vi "NicmosController.vi"() -> ()   [LabVIEW 2009]
uses:
  Controls/NICMOS.MASKBANKS.ctl
  Controls/NICMOS.COMMANDBASIC.ctl
  Controls/NICMOS.STATE.ctl
  Controls/NICMOS.FILTERLIST.ctl
  Controls/NICMOS.FILTER.ctl
  Controls/NICMOS.COMMAND.ctl
  Controls/NICMOS.READOUT.ctl
  Controls/NICMOS.FILTERCOMMAND.ctl
  Controls/NICMOS.TEMPERATURE.ctl
  NicmosGlobal.vi
panel:
  out "ACQ":i32
  in  "FilterList":T1=["DARK1", "J", "DARK3", "H", "DARK5", "K'", "BrG", "K203", "K215", "K222", "K239", "DARK12"]
  out "error out":errorcluster
  out "Index":i32
  out "STATE":T3
  out "COMMANDBASIC":T4=enum."QUIT"
  in  "VISA":string="COM31"
  in  "PROCESS":string="NICMOS"
  in  "MaskBanks":T5=[{"MaskList"=[{"X"=6, "Y"=6, "NX"=1, "NY"=1}], "Reform X"=1, "Reform Y"=1}, {"MaskList"=[{"X"=2, "Y"=2, "NX"=9, "NY"=9}], "Reform X"=9, "Reform Y"=9}, {"MaskList"=[{"X"=48, "Y"=38, "NX"=1, "NY"=8}], "Reform X"=1, "Reform Y"=8}, {"MaskList"=[{"X"=44, "Y"=38, "NX"=8, "NY"=8}], "Reform X"=8, "Reform Y"=8}, {"MaskList"=[{"X"=14, "Y"=7, "NX"=35, "NY"=8}], "Reform X"=35, "Reform Y"=8}, {"MaskList"=[{"X"=2, "Y"=2, "NX"=100, "NY"=100}], "Reform X"=100, "Reform Y"=100}]
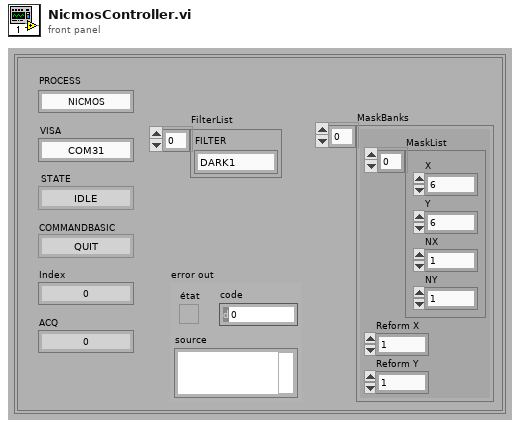
[diagram p1: front panel]
types:
  T1 = typedef "NICMOS.FILTERLIST.ctl" = T2[]
  T2 = typedef "NICMOS.FILTER.ctl" = string
  T3 = typedef "NICMOS.STATE.ctl" = enum16{"IDLE", "WRITING BANKS", "SETTING FILTER", "HOMING FILTER", "QUERYING TEMP", "CONFIGURING", "STARTING", "RUNNING", "HALTING", "STOPPED"}
  T4 = typedef "NICMOS.COMMANDBASIC.ctl" = enum16{"WRITE BANKS", "SET FILTER", "HOME FILTER", "QUERY TEMP", "CONFIGURE", "START", "ACQUISITION", "STOP", "QUIT"}
  T5 = typedef "NICMOS.MASKBANKS.ctl" = cluster{"MaskList":cluster{"X":i32, "Y":i32, "NX":i32, "NY":i32}[], "Reform X":i32, "Reform Y":i32}[]
  T6 = typedef "NicmosSynchronization.ctl" = cluster{"COMMAND":T7, "STATE":T8, "DATA":T9, "ACQUISITION":T10, "RAW":T11, "TEMPERATURE":T12, "READOUT":T13, "FILTER":T14, "MASKBANKS":T15}
  T7 = typedef "NICMOS.COMMAND.QUEUE.ctl" = refnum<queue>
  T8 = typedef "NICMOS.STATE.NOTIFIER.ctl" = refnum<notifier>
  T9 = typedef "NICMOS.DATA.NOTIFIER.ctl" = refnum<notifier>
  T10 = typedef "NICMOS.DATA.QUEUE.ctl" = refnum<queue>
  T11 = typedef "NICMOS.RAW.NOTIFIER.ctl" = refnum<notifier>
  T12 = typedef "NICMOS.TEMPERATURE.NOTIFIER.ctl" = refnum<notifier>
  T13 = typedef "NICMOS.READOUT.NOTIFIER.ctl" = refnum<notifier>
  T14 = typedef "NICMOS.FILTER.NOTIFIER.ctl" = refnum<notifier>
  T15 = typedef "NICMOS.MASKBANKS.NOTIFIER.ctl" = refnum<notifier>
  T16 = typedef "NICMOS.COMMAND.ctl" = cluster{"Command":T4, "READOUT":T17, "FILTERCOMMAND":T18, "ACQUISITION":i32, "Done":refnum<k4>}
  T17 = typedef "NICMOS.READOUT.ctl" = cluster{"Readout":i32, "Deglitch":i32, "Framerate":dbl[unit], "Bank":i32}
  T18 = typedef "NICMOS.FILTERCOMMAND.ctl" = cluster{"FILTER":T2, "INIT":bool}
  T19 = typedef "NICMOS.TEMPERATURE.ctl" = cluster{"T1":dbl, "T2":dbl}
  T20 = typedef "NICMOS.RAW.ctl" = u16[][][]
  T21 = typedef "NICMOS.DATA.ctl" = cluster{"DATA":i32[][][], "INDEX":i32}
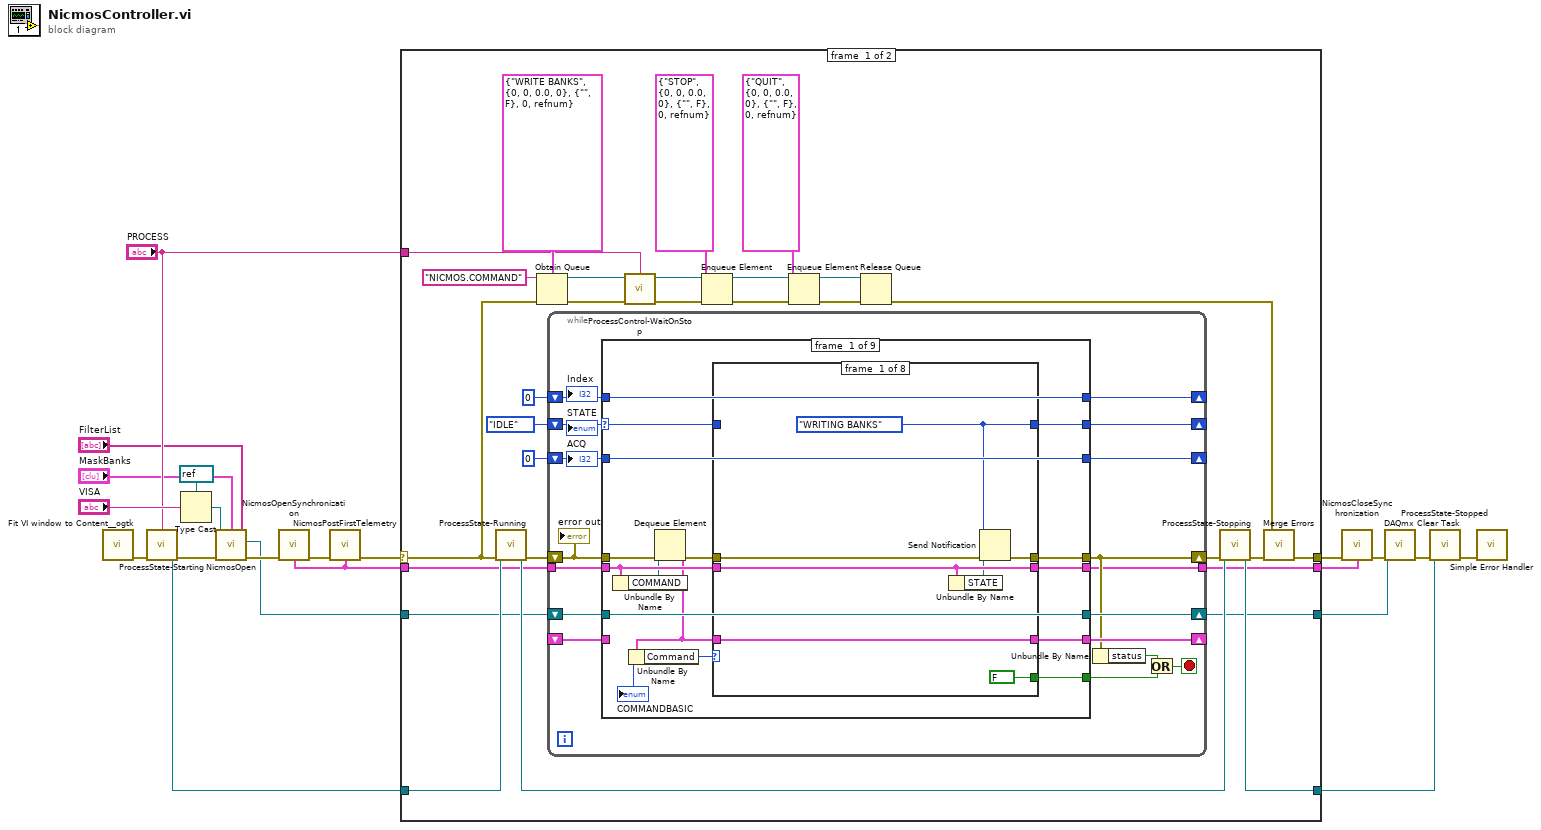
[diagram p0: block diagram]
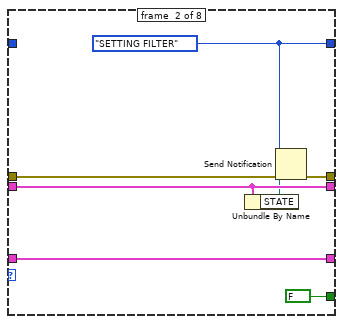
[diagram p2: hidden frame]
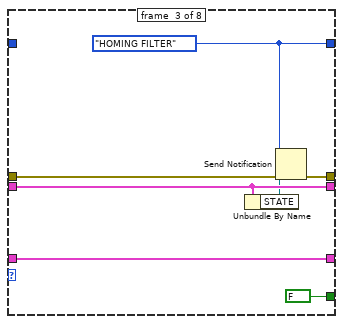
[diagram p3: hidden frame]
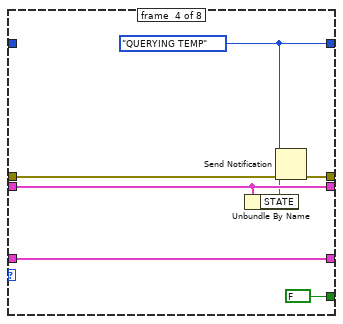
[diagram p4: hidden frame]
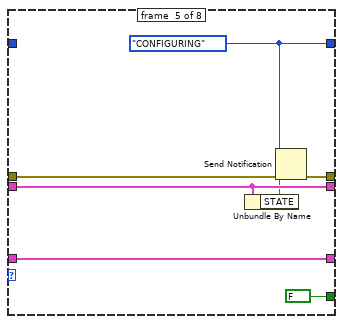
[diagram p5: hidden frame]
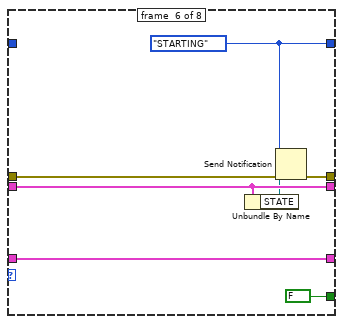
[diagram p6: hidden frame]
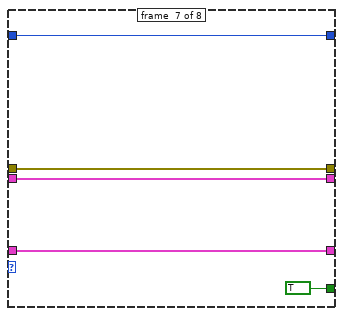
[diagram p7: hidden frame]
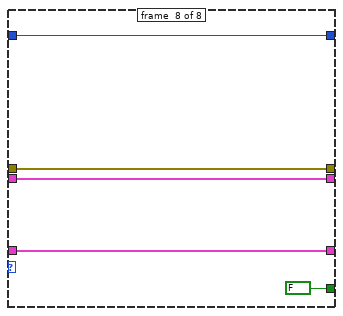
[diagram p8: hidden frame]
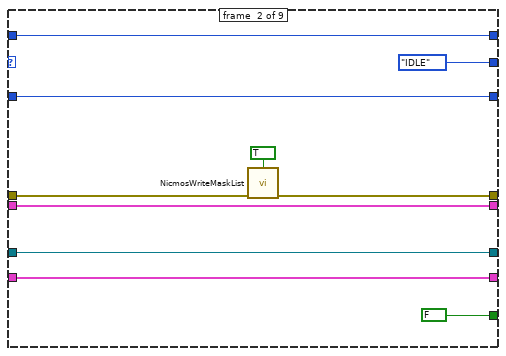
[diagram p9: hidden frame]
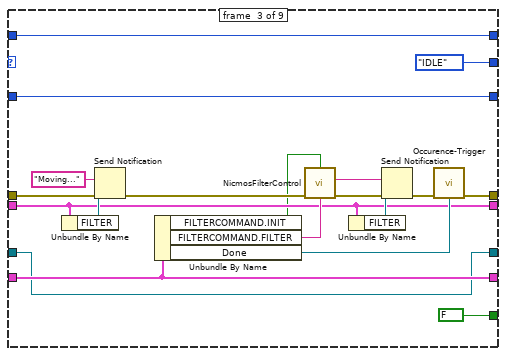
[diagram p10: hidden frame]
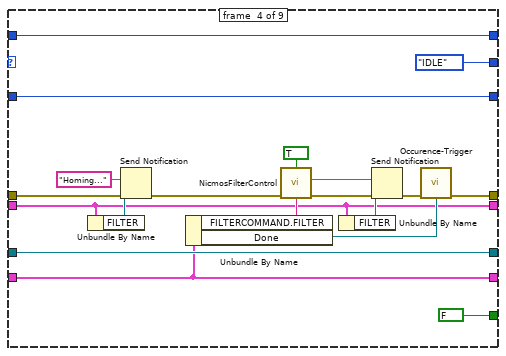
[diagram p11: hidden frame]
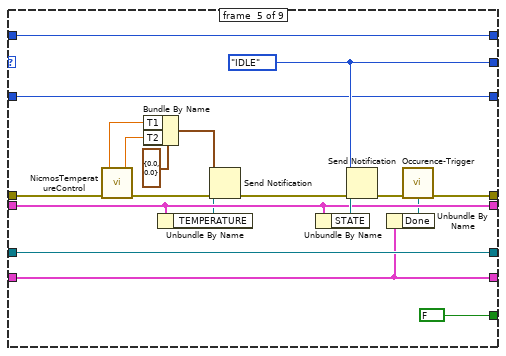
[diagram p12: hidden frame]
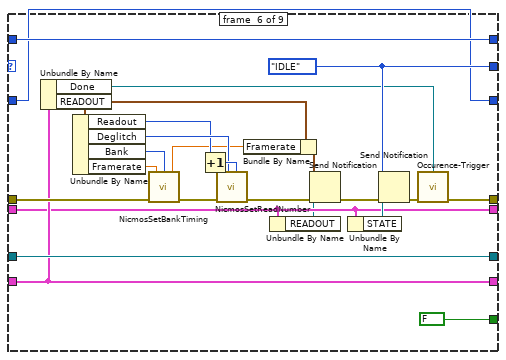
[diagram p13: hidden frame]
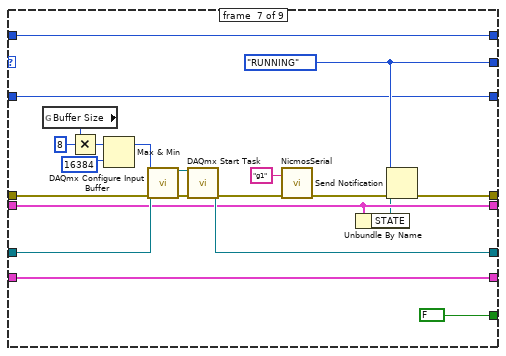
[diagram p14: hidden frame]
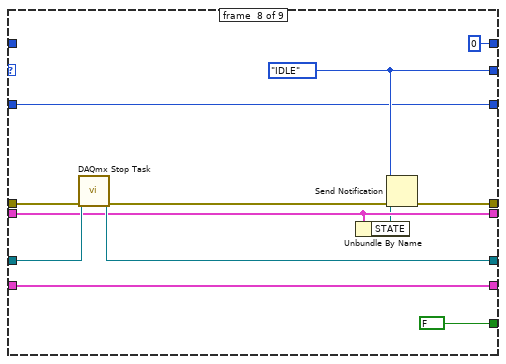
[diagram p15: hidden frame]
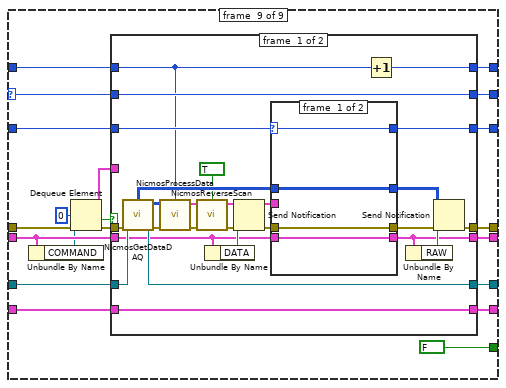
[diagram p16: hidden frame]
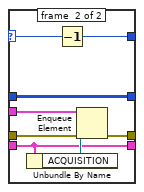
[diagram p17: hidden frame]
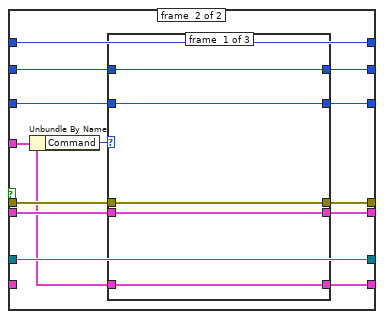
[diagram p18: hidden frame]
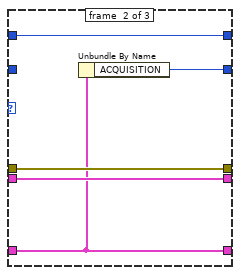
[diagram p19: hidden frame]
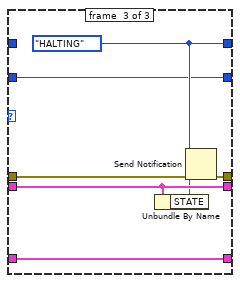
[diagram p20: hidden frame]
diagram:
  n1 = call <userlib>:"Fit VI window to Content__ogtk.vi"() -> ("error out"=w21:errorcluster)  [unwired: 6 in, 1 out]
  n2 = call "ProcessState-Starting.vi"("PROCESS"="PROCESS", "error in (no error)"=w21) -> ("ProcessStateNotifier"=w15:refnum<notifier>, "error in (no error)"=w20:errorcluster)  [unwired: 6 in]
  n3 = Type Cast(type=refnum<visa-resource-name> refnum ("COM Port"), x="VISA") -> (*(type *) &x=w17:refnum<visa-resource-name>)
  n4 = call "NicmosOpen.vi"("FilterList"="FilterList", "MASKBANKS"="MaskBanks", "NICMOS Port"=w17, "error in (no error)"=w20) -> ("NICMOS task out"=w10:refnum<k21>, "error out"=w16:errorcluster)  [unwired: 4 in]
  n5 = call "NicmosOpenSynchronization.vi"("error out"=w16) -> ("Synchronization"=w6:T6, "error in (no error)"=w7:errorcluster)  [unwired: 7 in]
  n6 = call "NicmosPostFirstTelemetry.vi"("Synchronization"=w6, "error in (no error)"=w7) -> ("error out"=w1:errorcluster)  [unwired: 7 in]
  n7 = case shown="No Error" w1 {
    selector: w1 -> [w22 w345]
    tunnel: w15 -> [w46 w342]
    tunnel: [w44 w342] -> w14
    tunnel: "PROCESS" -> [w40 _]
    tunnel: [w32 w345] -> w12
    tunnel: w10 -> [w28 w343]
    tunnel: [w27 w344] -> w9
    tunnel: w6 -> [w26 w344]
    tunnel: [w25 w343] -> w4
    frame #0 {
      n8 = call "ProcessState-Running.vi"("ProcessStateNotifier in"=w46, "error in (no error)"=w22) -> ("ProcessStateNotifier out"=w45:refnum<notifier>, "error out"=w48:errorcluster)  [unwired: 6 in]
      n9 = Obtain Queue(name (unnamed)="NICMOS.COMMAND" ("nom (aucun)"), element data type=T16 {"Command"=enum."WRITE BANKS", "READOUT"={"Readout"=0, "Deglitch"=0, "Framerate"=0.0, "Bank"=0}, "FILTERCOMMAND"={"FILTER"="", "INIT"=FALSE}, "ACQUISITION"=0, "Done"=refnum} ("NicmosCommand"), error in (no error)=w22) -> (queue out=w39:refnum<queue>, error out=w42:errorcluster)  [unwired: 2 in, 1 out]
      n10 = while {
        shift-right: [w58] -> w47
        shift-left: w48 -> [w66]
        shift-right: [w52] -> _
        shift-left: NICMOS.STATE."IDLE" ("STATE") -> [w61]
        shift-right: [w65] -> _
        shift-left: _ -> [w64]
        shift-right: [w63] -> _
        shift-left: 0 -> [w62]
        shift-right: [w60] -> w25
        shift-left: w28 -> [w59]
        tunnel: w26 -> [w54]
        tunnel: [w53] -> w27
        shift-right: [w50] -> _
        shift-left: 0 -> [w51]
        stop <- w55 stop-if-true
        n11 = case shown="\"RUNNING\"" w61 {
          selector: w61 -> [w80 _ _ _ _ _ _ _ w271]
          tunnel: w66 -> [w81 w136 w152 w168 w198 w220 w232 w252 w272]
          tunnel: [w79 NICMOS.STATE."IDLE" ("STATE") NICMOS.STATE."IDLE" ("STATE") NICMOS.STATE."IDLE" ("STATE") w190 w215 w225 w247 w268] -> w52
          tunnel: [w77 w135 w146 w174 w192 w201 w243 w255 w275] -> w58
          tunnel: [w76 FALSE FALSE FALSE FALSE FALSE FALSE FALSE FALSE] -> w56
          tunnel: [w74 w143 w159 w176 w194 w214 w241 w253 w269] -> w65
          tunnel: w64 -> [_ w143 w159 w176 w194 w214 w241 w253 w258]
          tunnel: w62 -> [w73 w138 w161 w179 w196 w218 w231 _ w267]
          tunnel: [w73 w138 w161 w179 w196 w218 w231 0 w266] -> w63
          tunnel: [w72 w142 w144 w178 w195 w217 w229 w250 w265] -> w60
          tunnel: w59 -> [w72 w142 w144 w178 w195 w217 w230 w251 w264]
          tunnel: w54 -> [w71 w141 w150 w162 w189 w207 w227 w249 w261]
          tunnel: [w69 w141 w150 w162 w189 w207 w227 w249 w263] -> w53
          tunnel: w51 -> [w67 w134 w156 w171 w180 w199 w223 w245 w259]
          tunnel: [w67 w134 w156 w171 w180 w199 w223 w245 w256] -> w50
          frame #0 {
            n12 = Unbundle By Name(w71) -> ("COMMAND"=w68:T7)
            n13 = Dequeue Element(queue=w68, error in (no error)=w81) -> (element=w70:T16, error out=w78:errorcluster)  [unwired: 1 in, 2 out]
            n14 = Unbundle By Name(w70) -> ("Command"=w75:T4)
            "COMMANDBASIC" <- w75
            n15 = case shown="\"QUERY TEMP\"" w75 {
              tunnel: w80 -> [_ _ _ _ _ _ w127 w133]
              tunnel: [w83 w90 w97 w105 w112 w118 w127 w133] -> w79
              tunnel: w78 -> [w84 w91 w98 w104 w111 w119 w128 w132]
              tunnel: [w86 w93 w100 w109 w116 w123 w128 w132] -> w77
              tunnel: [FALSE FALSE FALSE FALSE FALSE FALSE TRUE FALSE] -> w76
              tunnel: w70 -> [w88 w95 w102 w107 w114 w121 w125 w130]
              tunnel: [w88 w95 w102 w107 w114 w121 w125 w130] -> w74
              tunnel: w71 -> [w85 w92 w99 w106 w113 w120 w124 w129]
              tunnel: [w85 w92 w99 w106 w113 w120 w124 w129] -> w69
              frame #0 {
                w83 = NICMOS.STATE."WRITING BANKS" ("STATE")
                n16 = Unbundle By Name(w85) -> ("STATE"=w82:T8)
                n17 = Send Notification(notification=w83, notifier=w82, error in (no error)=w84) -> (error out=w86:errorcluster)  [unwired: 1 out]
              }
              frame #1 {
                w90 = NICMOS.STATE."SETTING FILTER" ("STATE")
                n18 = Unbundle By Name(w92) -> ("STATE"=w89:T8)
                n19 = Send Notification(notification=w90, notifier=w89, error in (no error)=w91) -> (error out=w93:errorcluster)  [unwired: 1 out]
              }
              frame #2 {
                w97 = NICMOS.STATE."HOMING FILTER" ("STATE")
                n20 = Unbundle By Name(w99) -> ("STATE"=w96:T8)
                n21 = Send Notification(notification=w97, notifier=w96, error in (no error)=w98) -> (error out=w100:errorcluster)  [unwired: 1 out]
              }
              frame #3 {
                w105 = NICMOS.STATE."QUERYING TEMP" ("STATE")
                n22 = Unbundle By Name(w106) -> ("STATE"=w103:T8)
                n23 = Send Notification(notification=w105, notifier=w103, error in (no error)=w104) -> (error out=w109:errorcluster)  [unwired: 1 out]
              }
              frame #4 {
                w112 = NICMOS.STATE."CONFIGURING" ("STATE")
                n24 = Unbundle By Name(w113) -> ("STATE"=w110:T8)
                n25 = Send Notification(notification=w112, notifier=w110, error in (no error)=w111) -> (error out=w116:errorcluster)  [unwired: 1 out]
              }
              frame #5 {
                w118 = NICMOS.STATE."STARTING" ("STATE")
                n26 = Unbundle By Name(w120) -> ("STATE"=w117:T8)
                n27 = Send Notification(notification=w118, notifier=w117, error in (no error)=w119) -> (error out=w123:errorcluster)  [unwired: 1 out]
              }
              frame #6 {
              }
              frame #7 {
              }
            }
          }
          frame #1 {
            n28 = call "NicmosWriteMaskList.vi"("Force Write Mask"=TRUE, "error in"=w136) -> ("error out"=w135:errorcluster)  [unwired: 7 in]
          }
          frame #2 {
            n29 = Unbundle By Name(w150) -> ("FILTER"=w153:T14)
            n30 = Send Notification(notification=T2 "Moving...", notifier=w153, error in (no error)=w152) -> (error out=w151:errorcluster)  [unwired: 1 out]
            n31 = Unbundle By Name(w159) -> ("FILTERCOMMAND.INIT"=w145:bool, "FILTERCOMMAND.FILTER"=w154:T2, "Done"=w157:refnum<k4>)
            n32 = call "NicmosFilterControl.vi"("Initialize"=w145, "FILTER"=w154, "error in (no error)"=w151) -> ("error out"=w148:errorcluster)  [unwired: 6 in]
            n33 = Unbundle By Name(w150) -> ("FILTER"=w155:T14)
            n34 = Send Notification(notification=w154, notifier=w155, error in (no error)=w148) -> (error out=w147:errorcluster)  [unwired: 1 out]
            n35 = call "Occurence-Trigger.vi"("Done"=w157, "error in (no error)"=w147) -> ("error out"=w146:errorcluster)  [unwired: 7 in]
          }
          frame #3 {
            n36 = Unbundle By Name(w162) -> ("FILTER"=w169:T14)
            n37 = Send Notification(notification=T2 "Homing...", notifier=w169, error in (no error)=w168) -> (error out=w167:errorcluster)  [unwired: 1 out]
            n38 = Unbundle By Name(w176) -> ("FILTERCOMMAND.FILTER"=w163:T2, "Done"=w173:refnum<k4>)
            n39 = call "NicmosFilterControl.vi"("Initialize"=TRUE, "FILTER"=w163, "error in (no error)"=w167) -> ("error out"=w165:errorcluster)  [unwired: 6 in]
            n40 = Unbundle By Name(w162) -> ("FILTER"=w166:T14)
            n41 = Send Notification(notification=w163, notifier=w166, error in (no error)=w165) -> (error out=w164:errorcluster)  [unwired: 1 out]
            n42 = call "Occurence-Trigger.vi"("Done"=w173, "error in (no error)"=w164) -> ("error out"=w174:errorcluster)  [unwired: 7 in]
          }
          frame #4 {
            w190 = NICMOS.STATE."IDLE" ("STATE")
            n43 = call "NicmosTemperatureControl.vi"("error in (no error)"=w198) -> ("T2"=w183:dbl, "T1"=w184:dbl, "error out"=w188:errorcluster)  [unwired: 4 in]
            n44 = Bundle By Name(cluster=T19 {"T1"=0.0, "T2"=0.0} ("notification"), "T1"=w184, "T2"=w183) -> (w185:T19)
            n45 = Unbundle By Name(w189) -> ("TEMPERATURE"=w182:T12)
            n46 = Send Notification(notification=w185, notifier=w182, error in (no error)=w188) -> (error out=w187:errorcluster)  [unwired: 1 out]
            n47 = Unbundle By Name(w189) -> ("STATE"=w191:T8)
            n48 = Send Notification(notification=w190, notifier=w191, error in (no error)=w187) -> (error out=w193:errorcluster)  [unwired: 1 out]
            n49 = Unbundle By Name(w194) -> ("Done"=w181:refnum<k4>)
            n50 = call "Occurence-Trigger.vi"("Done"=w181, "error in (no error)"=w193) -> ("error out"=w192:errorcluster)  [unwired: 7 in]
          }
          frame #5 {
            w215 = NICMOS.STATE."IDLE" ("STATE")
            n51 = Unbundle By Name(w214) -> ("Done"=w200:refnum<k4>, "READOUT"=w209:T17)
            n52 = Unbundle By Name(w209) -> ("Readout"=w210:i32, "Deglitch"=w211:i32, "Bank"=w212:i32, "Framerate"=w213:dbl[unit])
            n53 = call "NicmosSetBankTiming.vi"("error in"=w220, "Bank Number"=w212, "Frame rate"=w213) -> ("error out"=w219:errorcluster, "Frame rate (out)"=w208:dbl[unit])  [unwired: 2 in]
            n54 = Increment(x=w210) -> (x+1=w221:i32)
            n55 = call "NicmosSetReadNumber.vi"("Read Number"=w221, "Degitch"=w211, "error in"=w219) -> ("error out"=w205:errorcluster)  [unwired: 5 in]
            n56 = Bundle By Name(cluster=w209, "Framerate"=w208) -> (w203:T17)
            n57 = Unbundle By Name(w207) -> ("READOUT"=w206:T13)
            n58 = Send Notification(notification=w203, notifier=w206, error in (no error)=w205) -> (error out=w204:errorcluster)  [unwired: 1 out]
            n59 = Unbundle By Name(w207) -> ("STATE"=w216:T8)
            n60 = Send Notification(notification=w215, notifier=w216, error in (no error)=w204) -> (error out=w202:errorcluster)  [unwired: 1 out]
            n61 = call "Occurence-Trigger.vi"("Done"=w200, "error in (no error)"=w202) -> ("error out"=w201:errorcluster)  [unwired: 7 in]
          }
          frame #6 {
            w225 = NICMOS.STATE."RUNNING" ("STATE")
            n62 = global read "NicmosGlobal.vi" "Buffer Size"() -> (w240:u32)
            n63 = Multiply(x=w240, y=u32 8) -> (x*y=w238:u32)
            n64 = Max & Min(x=w238, y=u32 16384) -> (max(x,y)=w228:u32)  [unwired: 1 out]
            n65 = call <vilib>:"DAQmx Configure Input Buffer.vi"("task/channels in"=w230, "buffer size (in samples per channel)"=w228, "error in"=w232) -> ("task out"=w237:refnum<k21>, "error out"=w236:errorcluster)  [unwired: 11 in]
            n66 = call <vilib>:"DAQmx Start Task.vi"("task/channels in"=w237, "error in"=w236) -> ("task out"=w229:refnum<k21>, "error out"=w235:errorcluster)  [unwired: 12 in]
            n67 = call "NicmosSerial.vi"("error in"=w235, "Command"="g1") -> ("error out"=w226:errorcluster)  [unwired: 3 in, 1 out]
            n68 = Unbundle By Name(w227) -> ("STATE"=w224:T8)
            n69 = Send Notification(notification=w225, notifier=w224, error in (no error)=w226) -> (error out=w243:errorcluster)  [unwired: 1 out]
          }
          frame #7 {
            w247 = NICMOS.STATE."IDLE" ("STATE")
            n70 = call <vilib>:"DAQmx Stop Task.vi"("task/channels in"=w251, "error in"=w252) -> ("task out"=w250:refnum<k21>, "error out"=w248:errorcluster)  [unwired: 12 in]
            n71 = Unbundle By Name(w249) -> ("STATE"=w246:T8)
            n72 = Send Notification(notification=w247, notifier=w246, error in (no error)=w248) -> (error out=w255:errorcluster)  [unwired: 1 out]
          }
          frame #8 {
            n73 = Unbundle By Name(w261) -> ("COMMAND"=w260:T7)
            n74 = Dequeue Element(queue=w260, timeout in ms (-1)=0 ("timeout en ms (-1)"), error in (no error)=w272) -> (element=w257:T16, timed out?=w270:bool, error out=w273:errorcluster)  [unwired: 1 out]
            n75 = case shown="True" w270 {
              tunnel: [w284 w324] -> w275
              tunnel: w273 -> [w299 w323]
              tunnel: w271 -> [w297 w319]
              tunnel: [w298 w322] -> w269
              tunnel: w258 -> [w298 _]
              tunnel: [w297 w320] -> w268
              tunnel: w257 -> [_ w313]
              tunnel: w267 -> [w277 w318]
              tunnel: [w296 w318] -> w266
              tunnel: [w290 w317] -> w265
              tunnel: w264 -> [w295 w317]
              tunnel: w261 -> [w287 w316]
              tunnel: [w280 w315] -> w263
              tunnel: w259 -> [w282 w314]
              tunnel: [w281 w312] -> w256
              frame #0 {
                n76 = call "NicmosGetDataDAQ.vi"("task/channels in"=w295, "error out"=w299) -> ("task out"=w290:refnum<k21>, "NICMOS.RAW"=w279:T20, "error in (no error)"=w294:errorcluster)  [unwired: 5 in]
                n77 = call "NicmosProcessData.vi"("Index"=w277, "Data In"=w279, "error out"=w294) -> ("Data Out"=w293:T21, "error in (no error)"=w292:errorcluster)  [unwired: 5 in]
                n78 = call "NicmosReverseScan.vi"("Scan"=w293, "Reverse"=TRUE, "error out"=w292) -> ("Reversed Scan"=w285:T21, "error in (no error)"=w291:errorcluster)  [unwired: 5 in]
                n79 = Unbundle By Name(w287) -> ("DATA"=w288:T9)
                n80 = Send Notification(notification=w285, notifier=w288, error in (no error)=w291) -> (error out=w286:errorcluster)  [unwired: 1 out]
                n81 = case shown="1, Default" w282 {
                  selector: w282 -> [w301 w307]
                  tunnel: w287 -> [w302 w305]
                  tunnel: w286 -> [w303 w310]
                  tunnel: w285 -> [_ w309]
                  tunnel: [w303 w308] -> w283
                  tunnel: [w301 w306] -> w281
                  tunnel: [w302 w305] -> w280
                  tunnel: w279 -> [w300 w304]
                  tunnel: [w300 w304] -> w278
                  frame #0 {
                  }
                  frame #1 {
                    n82 = Unbundle By Name(w305) -> ("ACQUISITION"=w311:T10)
                    n83 = Decrement(x=w307) -> (x-1=w306:i32)
                    n84 = Enqueue Element(queue=w311, element=w309, error in (no error)=w310) -> (error out=w308:errorcluster)  [unwired: 1 in, 2 out]
                  }
                }
                n85 = Increment(x=w277) -> (x+1=w296:i32)
                n86 = Unbundle By Name(w280) -> ("RAW"=w289:T11)
                n87 = Send Notification(notification=w278, notifier=w289, error in (no error)=w283) -> (error out=w284:errorcluster)  [unwired: 1 out]
              }
              frame #1 {
                n88 = Unbundle By Name(w313) -> ("Command"=w321:T4)
                n89 = case shown="\"ACQUISITION\"" w321 {
                  tunnel: [w329 w333 w341] -> w324
                  tunnel: w323 -> [w329 w333 w337]
                  tunnel: w313 -> [w328 w331 w340]
                  tunnel: [w328 w331 w340] -> w322
                  tunnel: [w327 w332 w338] -> w320
                  tunnel: w319 -> [w327 w332 _]
                  tunnel: w316 -> [w326 w334 w339]
                  tunnel: [w326 w334 w339] -> w315
                  tunnel: w314 -> [w325 _ w335]
                  tunnel: [w325 w330 w335] -> w312
                  frame #0 {
                  }
                  frame #1 {
                    n90 = Unbundle By Name(w331) -> ("ACQUISITION"=w330:i32)
                  }
                  frame #2 {
                    w338 = NICMOS.STATE."HALTING" ("STATE")
                    n91 = Unbundle By Name(w339) -> ("STATE"=w336:T8)
                    n92 = Send Notification(notification=w338, notifier=w336, error in (no error)=w337) -> (error out=w341:errorcluster)  [unwired: 1 out]
                  }
                }
              }
            }
          }
        }
        n93 = Unbundle By Name(w58) -> ("status"=w57:bool)
        n94 = Or(x=w57, y=w56) -> (x .or. y?=w55:bool)
        "Index" <- w62
        "STATE" <- w61
        "error out" <- w66
        "ACQ" <- w51
      }
      n95 = call "ProcessControl-WaitOnStop.vi"("PROCESS"=w40, "error out"=w42) -> ("error in"=w41:errorcluster)  [unwired: 7 in]
      n96 = Enqueue Element(queue=w39, element=T16 {"Command"=enum."STOP", "READOUT"={"Readout"=0, "Deglitch"=0, "Framerate"=0.0, "Bank"=0}, "FILTERCOMMAND"={"FILTER"="", "INIT"=FALSE}, "ACQUISITION"=0, "Done"=refnum} ("élément"), error in (no error)=w41) -> (queue out=w36:refnum<queue>, error out=w37:errorcluster)  [unwired: 1 in, 1 out]
      n97 = Enqueue Element(queue=w36, element=T16 {"Command"=enum."QUIT", "READOUT"={"Readout"=0, "Deglitch"=0, "Framerate"=0.0, "Bank"=0}, "FILTERCOMMAND"={"FILTER"="", "INIT"=FALSE}, "ACQUISITION"=0, "Done"=refnum} ("élément"), error in (no error)=w37) -> (queue out=w34:refnum<queue>, error out=w35:errorcluster)  [unwired: 1 in, 1 out]
      n98 = Release Queue(queue=w34, error in (no error)=w35) -> (error out=w31:errorcluster)  [unwired: 1 in, 2 out]
      n99 = call "ProcessState-Stopping.vi"("ProcessStateNotifier in"=w45, "error in (no error)"=w47) -> ("ProcessStateNotifier out"=w44:refnum<notifier>, "error out"=w33:errorcluster)  [unwired: 6 in]
      n100 = call <vilib>:"Merge Errors.vi"("error in 3 (no error)"=w33, "error in 1 (no error)"=w31) -> ("error out"=w32:errorcluster)  [unwired: 5 in]
    }
    frame #1 {
    }
  }
  n101 = call "NicmosCloseSynchronization.vi"("Synchronization"=w9, "error out"=w12) -> ("error in (no error)"=w5:errorcluster)  [unwired: 7 in]
  n102 = call <vilib>:"DAQmx Clear Task.vi"("task in"=w4, "error in"=w5) -> ("error out"=w3:errorcluster)  [unwired: 13 in]
  n103 = call "ProcessState-Stopped.vi"("ProcessStateNotifier in"=w14, "error in (no error)"=w3) -> ("error out"=w2:errorcluster)  [unwired: 7 in]
  n104 = call <vilib>:"Simple Error Handler.vi"("error in (no error)"=w2) -> ()  [unwired: 4 in, 5 out]
